vi "F5xxx_wait_settle.vi"(8 "error in":errorcluster, 10 "ms to wait":i32=10000, 11 "VISA in":refnum<visa-resource-name>) -> (0 "error out":errorcluster, 3 "VISA out":refnum<visa-resource-name>)   [LabVIEW 2013]
uses:
  Fluke 5XXX Series Multicalibrators.lvlib
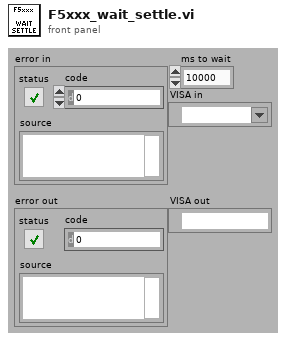
[diagram p1: front panel]
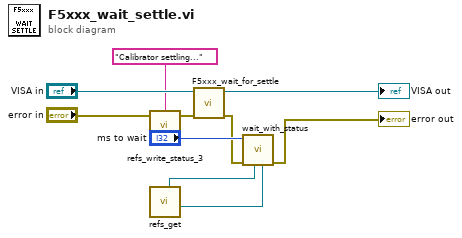
[diagram p0: block diagram]
diagram:
  n1 = call "refs_write_status_3.vi"("error in"="error in", "Value"="Calibrator settling...") -> ("error out"=w3:errorcluster)  [unwired: 2 in]
  n2 = call "refs_get.vi"() -> ("stat 3 ref"=w6:refnum<vi>, "btn stop ref"=w7:refnum<vi>)  [unwired: 5 in, 5 out]
  n3 = call "F5xxx_wait_for_settle.vi"("error in (no error)"=w3, "VISA Refnum in"="VISA in") -> ("error out"=w5:errorcluster, "VISA Refnum out"=→"VISA out":refnum<visa-resource-name>)  [unwired: 7 in, 1 out]
  n4 = call "wait_with_status.vi"("stat ref"=w6, "stop ref"=w7, "error in"=w5, "ms to wait"="ms to wait") -> ("error out"=→"error out":errorcluster)  [unwired: 7 in]
